vi "load DSF Configuration from file.vi"(7 "prompt (Choose or enter file path)":string, 8 "error in (no error)":errorcluster, 10 "file (use dialog)":path) -> (0 "error out":errorcluster, 2 "path":path, 3 "configuration cluster out":T1)   [LabVIEW 2017, in "DSF Configuration API v1.0.0.lvlib"]
uses:
  DSF Configuration API v1.0.0.lvlib
  Controls/dsf configuration file/1.0.0/dsf configuration.ctl
  Controls/dsf configuration file/1.0.0/version.ctl
  Controls/dsf configuration file/1.0.0/dsf plugin.ctl
  Controls/dsf configuration file/1.0.0/dsf timing.ctl
  Controls/dsf configuration file/1.0.0/dsf group.ctl
  Controls/dsf configuration file/1.0.0/dsf transfer.ctl
  Controls/dsf configuration file/1.0.0/dsf channel.ctl
  Controls/dsf configuration file/1.0.0/dsf settings.ctl
  Controls/dsf configuration file/1.0.0/dsf configuration file v1.0.0.lvlib
panel:
  # "dsf\nfile"
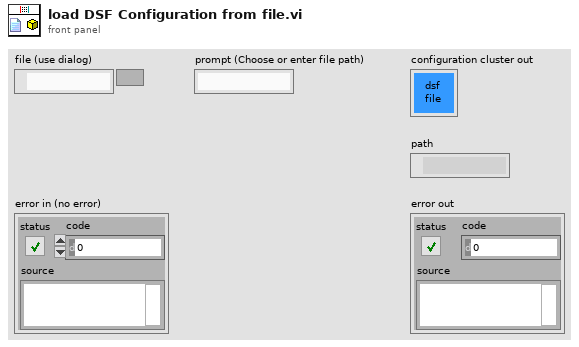
[diagram p1: front panel]
types:
  T1 = typedef "dsf configuration file v1.0.0.lvlib/dsf configuration.ctl" = cluster{"dsf":T2, "configuration":T2, "plugins":T3[], "groups":T5[], "transfers":T6[], "channels":T7[], "settings":T8[]}
  T2 = typedef "dsf configuration file v1.0.0.lvlib/version.ctl" = cluster{"major":u32, "minor":u32, "fix":u32, "build":string}
  T3 = typedef "dsf configuration file v1.0.0.lvlib/dsf plugin.ctl" = cluster{"id":string, "values":cluster{"type":string, "timing":T4, "group ids":string[], "settings id":string}}
  T4 = typedef "dsf configuration file v1.0.0.lvlib/dsf timing.ctl" = cluster{"decimation":i32, "offset":i32}
  T5 = typedef "dsf configuration file v1.0.0.lvlib/dsf group.ctl" = cluster{"id":string, "values":cluster{"direction":i32, "timing":T4, "transfer ids":string[], "settings id":string}}
  T6 = typedef "dsf configuration file v1.0.0.lvlib/dsf transfer.ctl" = cluster{"id":string, "values":cluster{"byte order":i32, "channel ids":string[], "settings id":string}}
  T7 = typedef "dsf configuration file v1.0.0.lvlib/dsf channel.ctl" = cluster{"id":string, "values":cluster{"count":i32, "offset":i32, "data type":i32, "resource path":string, "settings id":string}}
  T8 = typedef "dsf configuration file v1.0.0.lvlib/dsf settings.ctl" = cluster{"id":string, "values":cluster{"key":string, "value":string}[]}
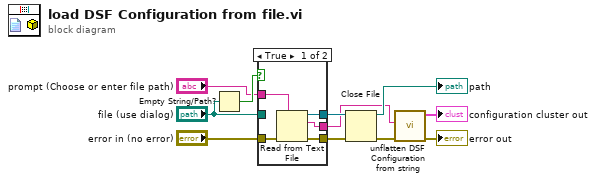
[diagram p0: block diagram]
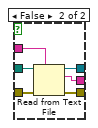
[diagram p2: hidden frame]
diagram:
  n1 = Empty String/Path?(string/path="file (use dialog)") -> (empty?=w9:bool)
  n2 = case shown="True" w9 {
    tunnel: "error in (no error)" -> [w16 w22]
    tunnel: [w15 w21] -> w1
    tunnel: [w14 w20] -> w11
    tunnel: "file (use dialog)" -> [_ w18]
    tunnel: "prompt (Choose or enter file path)" -> [w13 w19]
    tunnel: [w12 w17] -> w5
    frame True {
      n3 = Read from Text File(prompt (Open existing file)=w13, error in=w16) -> (refnum out=w14:refnum<file>, text=w12:string, error out=w15:errorcluster)  [unwired: 2 in, 1 out]
    }
    frame False {
      n4 = Read from Text File(prompt (Open existing file)=w19, file (use dialog)=w18, error in=w22) -> (refnum out=w20:refnum<file>, text=w17:string, error out=w21:errorcluster)  [unwired: 1 in, 1 out]
    }
  }
  n5 = Close File(refnum=w11, error in=w1) -> (path=→"path":path, error out=w3:errorcluster)
  n6 = call "unflatten DSF Configuration from string.vi"("error in"=w3, "String"=w5) -> ("error out"=→"error out":errorcluster, "dsf configuration out"=→"configuration cluster out":T1)  [unwired: 8 in]
